vi "624WPIAdjust Dashboard Window.vi"(8 "Width":i16, 9 "Height":i16, 10 "VI":refnum<vi>, 11 "Notifier in":refnum<notifier>) -> ()   [LabVIEW 2017]
uses:
  <vilib>/Utility/miscctls.llb/LVRectTypeDef.ctl
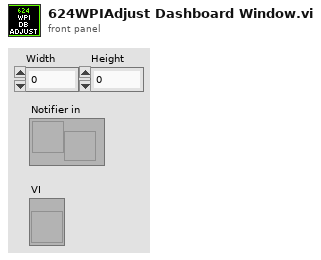
[diagram p1: front panel]
types:
  T1 = typedef "LVRectTypeDef.ctl" = cluster{"Left":i16, "Top":i16, "Right":i16, "Bottom":i16}
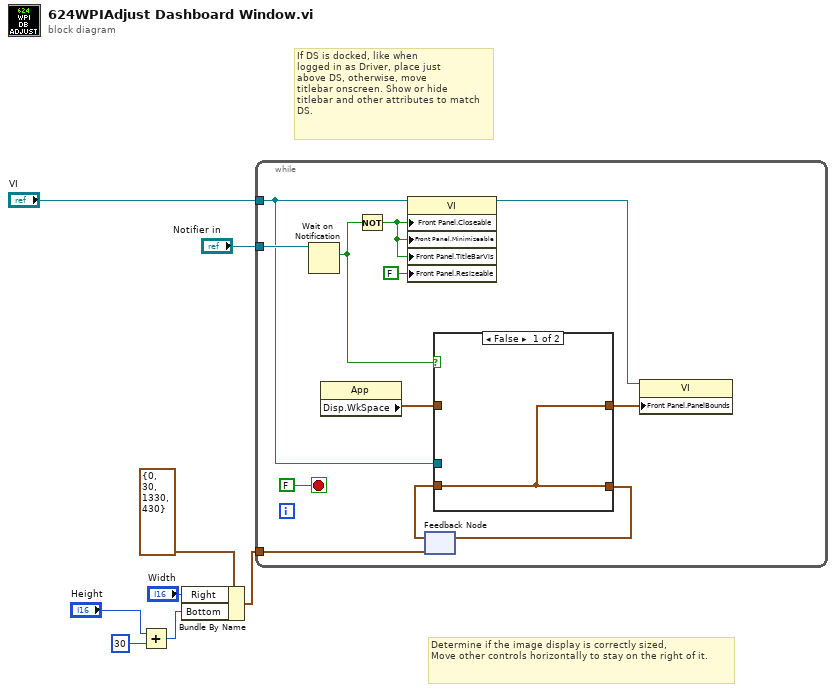
[diagram p0: block diagram]
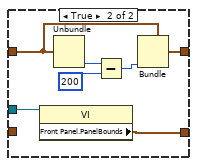
[diagram p2: hidden frame]
diagram:
  # "Determine if the image display is correctly sized,\nMove other controls horizontally to stay on the right of it."
  # "If DS is docked, like when\nlogged in as Driver, place just\nabove DS, otherwise, move\ntitlebar onscreen. Show or hide\ntitlebar and other attributes to match\nDS."
  n1 = Add(x="Height", y=i16 30) -> (x+y=w2:i16)
  n2 = Bundle By Name(cluster=T1 {"Left"=0, "Top"=30, "Right"=1330, "Bottom"=430} ("Front Panel.PanelBounds"), "Right"="Width", "Bottom"=w2) -> (w1:T1)
  n3 = while {
    tunnel: "Notifier in" -> [w19]
    tunnel: "VI" -> [w14]
    tunnel: w1 -> [w11]
    stop <- FALSE stop-if-true
    n4 = Wait on Notification(notifier=w19) -> (notification=w15:bool)  [unwired: 3 in, 3 out]
    n5 = property class="App"() -> ("Disp.WkSpace"=w18:T1)  [unwired: 2 in, 2 out]
    n6 = Not(x=w15) -> (.not. x?=w10:bool)
    n7 = property class="VI"(reference=w14, "Front Panel.Closeable"=w10, "Front Panel.Minimizeable"=w10, "Front Panel.TitleBarVis"=w10, "Front Panel.Resizeable"=FALSE ("Front Panel Window:Resizable")) -> (reference out=w17:refnum<vi>)  [unwired: 1 in, 1 out]
    n8 = feedback #1(w11) -> (w12:T1)
    n9 = case shown="False" w15 {
      tunnel: w18 -> [_ w24]
      tunnel: [w21 w25] -> w16
      tunnel: w14 -> [_ w23]
      tunnel: [w21 w22] -> w13
      tunnel: w12 -> [w21 _]
      frame False {
      }
      frame True {
        n10 = property class="VI"(reference=w23) -> ("Front Panel.PanelBounds"=w22:T1)  [unwired: 1 in, 2 out]
        n11 = Unbundle(w24) -> ("Bottom"=w28:i16)  [unwired: 3 out]
        n12 = Subtract(x=w28, y=200) -> (x-y=w26:i32)
        n13 = Bundle(cluster=w24, "Bottom"=w26) -> (w25:T1)  [unwired: 3 out]
      }
    }
    n14 = feedback-in #1(w13) -> ()
    n15 = property class="VI"(reference=w17, "Front Panel.PanelBounds"=w16) -> ()  [unwired: 1 in, 2 out]
  }
